vi "G#Debugger_ClearTree.vi"(0 "Front Panel":refnum<vi>, 1 "Tree":refnum<vi>, 5 "error in (no error)":errorcluster) -> (19 "error out":errorcluster)   [LabVIEW 2017, in "G#Debugger.lvlib"]
uses:
  G#Debugger.lvlib
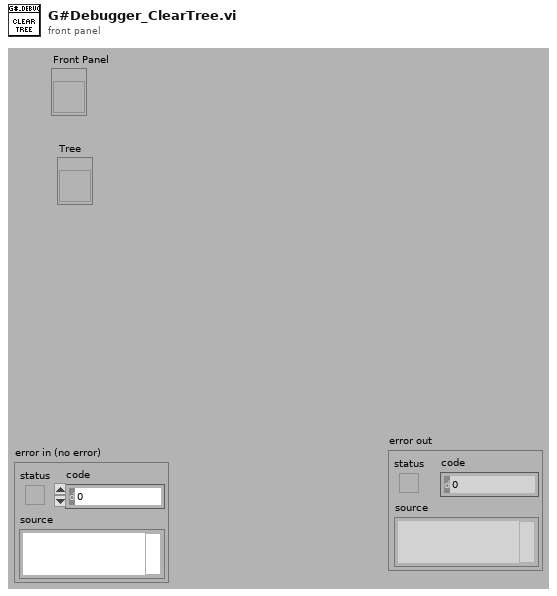
[diagram p1: front panel]
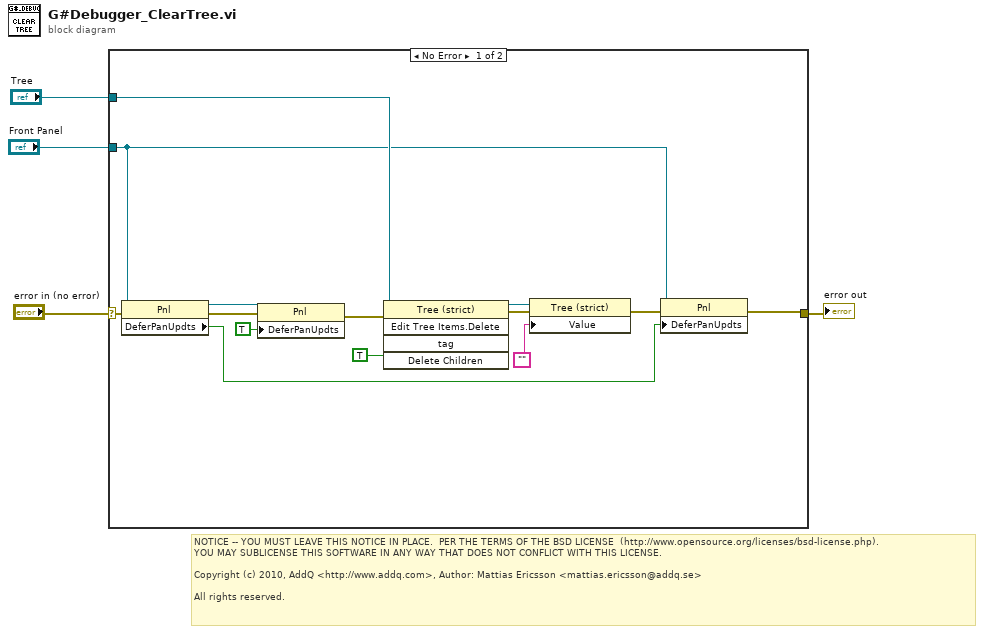
[diagram p0: block diagram]
diagram:
  # "NOTICE -- YOU MUST LEAVE THIS NOTICE IN PLACE.  PER THE TERMS OF THE BSD LICENSE  (http://www.opensource.org/licenses/bsd-license.php).\nYOU MAY SUBLICENSE THIS SOFTWARE IN ANY WAY THAT DOES NOT CONFLICT WITH THIS LICENSE.\n\nCopyright (c) 2010, AddQ <http://www.addq.com>, Author: Mattias Ericsson <mattias.ericsson@addq.se>\n\nAll rights reserved."
  n1 = case shown="No Error" "error in (no error)" {
    selector: "error in (no error)" -> [w9 w19]
    tunnel: [w10 w19] -> w3
    tunnel: "Tree" -> [w17 _]
    tunnel: "Front Panel" -> [w8 _]
    frame No Error {
      n2 = property class="Pnl"(reference=w8, error in=w9) -> (reference out=w6:refnum<vi>, error out=w7:errorcluster, "DeferPanUpdts"=w5:bool)
      n3 = property class="Pnl"(reference=w6, error in=w7, "DeferPanUpdts"=TRUE ("Defer Panel Updates")) -> (error out=w12:errorcluster)  [unwired: 1 out]
      n4 = invoke class="Tree (strict)" method="Edit Tree Items.Delete"(reference=w17, error in=w12, "Delete Children"=TRUE ("Delete Children?")) -> (reference out=w15:refnum<vi>, error out=w16:errorcluster)  [unwired: 2 in, 3 out]
      n5 = property class="Tree (strict)"(reference=w15, error in=w16, "Value"="") -> (error out=w11:errorcluster)  [unwired: 1 out]
      n6 = property class="Pnl"(reference=w8, error in=w11, "DeferPanUpdts"=w5) -> (error out=w10:errorcluster)  [unwired: 1 out]
    }
    frame Error {
    }
  }
  "error out" <- w3
